vi "cargarDatoReceta.vi"(11 "IndiceAUltimoValor\nAgregadoEnLaTabla":i32=1) -> ()   [LabVIEW 2014]
uses:
  claseReceta/claseReceta.lvclass
panel:
  out "dataReading":T1
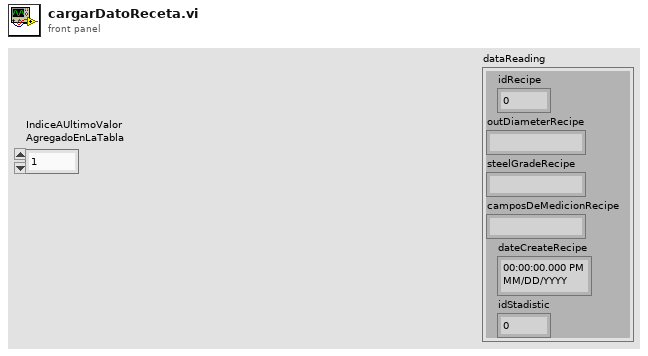
[diagram p1: front panel]
types:
  T1 = cluster{"idRecipe":dbl, "outDiameterRecipe":string, "steelGradeRecipe":string, "camposDeMedicionRecipe":string, "dateCreateRecipe":timestamp, "idStadistic":dbl}
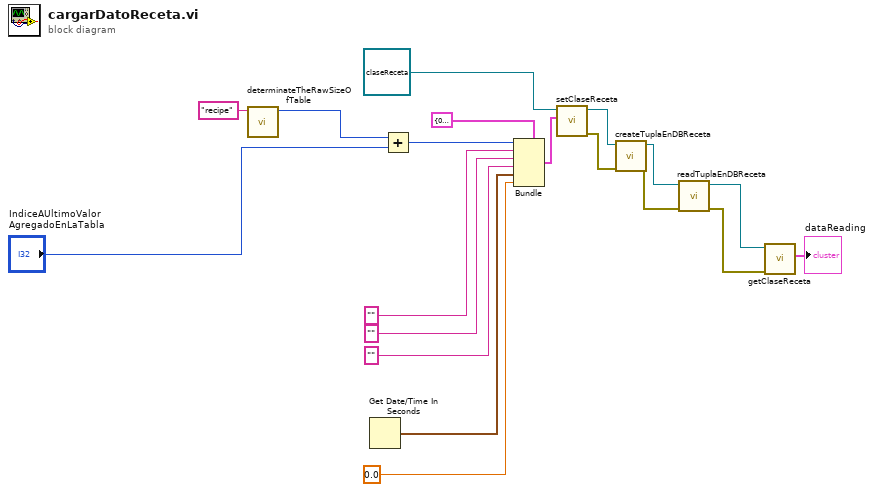
[diagram p0: block diagram]
diagram:
  n1 = call "determinateTheRawSizeOfTable.vi"("tableName"="recipe") -> ("sizeOfTableInNumberRaw"=w2:i32)  [unwired: 8 in, 1 out]
  n2 = Get Date/Time In Seconds() -> (seconds since 1Jan1904=w15:timestamp)
  n3 = Add(x=w2, y="IndiceAUltimoValor\nAgregadoEnLaTabla") -> (x+y=w16:i32)
  n4 = Bundle(cluster=T1 {"idRecipe"=0.0, "outDiameterRecipe"="", "steelGradeRecipe"="", "camposDeMedicionRecipe"="", "dateCreateRecipe"=timestamp(0 s since 1904-01-01), "idStadistic"=0.0} ("dataToSet"), "idRecipe"=w16, "outDiameterRecipe"="", "steelGradeRecipe"="", "camposDeMedicionRecipe"="", "dateCreateRecipe"=w15, "idStadistic"=0.0) -> (w10:T1)
  n5 = call "setClaseReceta.vi"("dataToSet"=w10, "claseReceta in"=refnum<class "claseReceta.lvclass"> refnum ("claseReceta.lvclass")) -> ("error out"=w8:errorcluster, "claseReceta out"=w9:refnum<class "claseReceta.lvclass">)  [unwired: 8 in]
  n6 = call "createTuplaEnDBReceta.vi"("error in"=w8, "claseReceta in"=w9) -> ("error out"=w6:errorcluster, "claseReceta out"=w7:refnum<class "claseReceta.lvclass">)  [unwired: 8 in]
  n7 = call "readTuplaEnDBReceta.vi"("error in"=w6, "claseReceta in"=w7) -> ("error out"=w4:errorcluster, "claseReceta out"=w5:refnum<class "claseReceta.lvclass">)  [unwired: 8 in]
  n8 = call "getClaseReceta.vi"("error in"=w4, "claseReceta in"=w5) -> ("dataReading"=→"dataReading":T1)  [unwired: 5 in, 2 out]
